vi "8 display.vi"(11 "Numeric":dbl) -> (1 "d":bool, 2 "c":bool, 3 "b":bool, 4 "e":bool, 5 "a":bool, 6 "f":bool, 7 "g":bool)   [LabVIEW 2019]
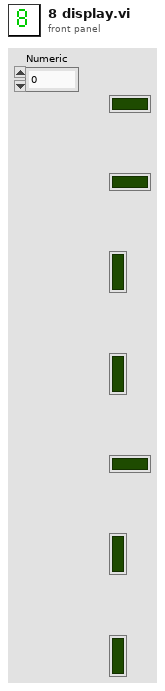
[diagram p1: front panel]
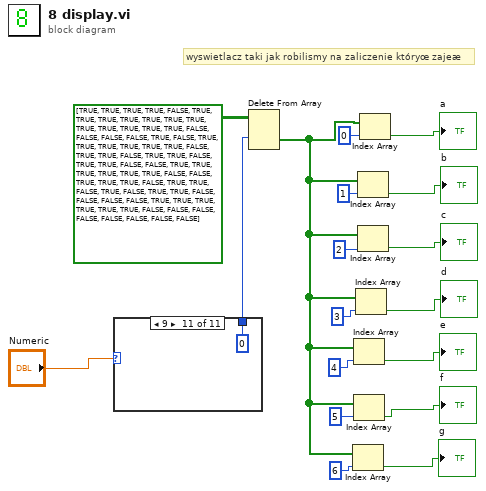
[diagram p0: block diagram]
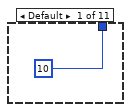
[diagram p2: hidden frame]
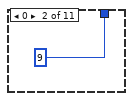
[diagram p3: hidden frame]
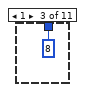
[diagram p4: hidden frame]
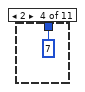
[diagram p5: hidden frame]
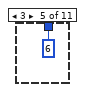
[diagram p6: hidden frame]
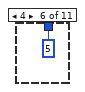
[diagram p7: hidden frame]
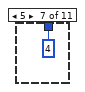
[diagram p8: hidden frame]
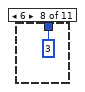
[diagram p9: hidden frame]
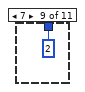
[diagram p10: hidden frame]
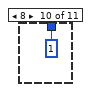
[diagram p11: hidden frame]
diagram:
  # "wyswietlacz taki jak robilismy na zaliczenie któryœ zajeæ"
  n1 = case shown="9" "Numeric" {
    tunnel: [10 9 ("index") 8 ("index") 7 ("index") 6 ("index") 5 ("index") 4 ("index") 3 ("index") 2 ("index") 1 ("index") 0 ("index")] -> w18
    frame Default {
    }
    frame 0 {
    }
    frame 1 {
    }
    frame 2 {
    }
    frame 3 {
    }
    frame 4 {
    }
    frame 5 {
    }
    frame 6 {
    }
    frame 7 {
    }
    frame 8 {
    }
    frame 9 {
    }
  }
  n2 = Delete From Array(array=bool[][] [[TRUE, TRUE, TRUE, TRUE, FALSE, TRUE, TRUE], [TRUE, TRUE, TRUE, TRUE, TRUE, TRUE, TRUE], [TRUE, TRUE, TRUE, FALSE, FALSE, FALSE, FALSE], [TRUE, FALSE, TRUE, TRUE, TRUE, TRUE, TRUE], [TRUE, FALSE, TRUE, TRUE, FALSE, TRUE, TRUE], [FALSE, TRUE, TRUE, FALSE, FALSE, TRUE, TRUE], [TRUE, TRUE, TRUE, TRUE, FALSE, FALSE, TRUE], [TRUE, TRUE, FALSE, TRUE, TRUE, FALSE, TRUE], [FALSE, TRUE, TRUE, FALSE, FALSE, FALSE, FALSE], [TRUE, TRUE, TRUE, TRUE, TRUE, TRUE, FALSE], [FALSE, FALSE, FALSE, FALSE, FALSE, FALSE, FALSE]], index (row)=w18) -> (deleted portion=w2:bool[])  [unwired: 2 in, 1 out]
  n3 = Index Array(array=w2, index=6) -> (element=→"g":bool)
  n4 = Index Array(array=w2, index=4) -> (element=→"e":bool)
  n5 = Index Array(array=w2, index=5) -> (element=→"f":bool)
  n6 = Index Array(array=w2, index=3) -> (element=→"d":bool)
  n7 = Index Array(array=w2, index=1) -> (element=→"b":bool)
  n8 = Index Array(array=w2, index=2) -> (element=→"c":bool)
  n9 = Index Array(array=w2, index=0) -> (element=→"a":bool)
